vi "MP-285 Get Position.vi"(5 "error in (no error)":errorcluster, 6 "VISA resource name":refnum<visa-resource-name>) -> (0 "error out":errorcluster, 1 "Output: Z axis (microns)":dbl format="%.2f", 2 "Output: Y axis (microns)":dbl format="%.2f", 3 "Output: X axis (microns)":dbl format="%.2f", 4 "VISA resource name out":refnum<visa-resource-name>)   [LabVIEW 2010]
uses:
  StageMG100204SutterMP285/StageMG100204SutterMP285.lvclass
panel:
  out "last element CR?":bool
  out "return count":u32
  out "Serial Read":string
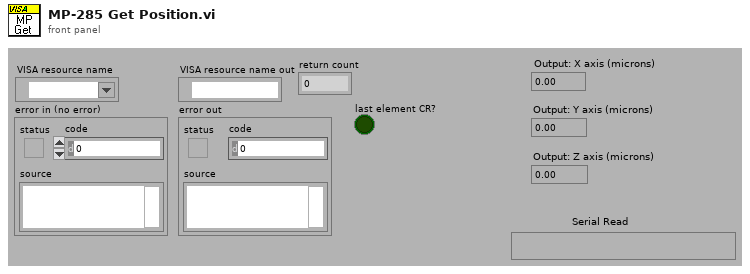
[diagram p1: front panel]
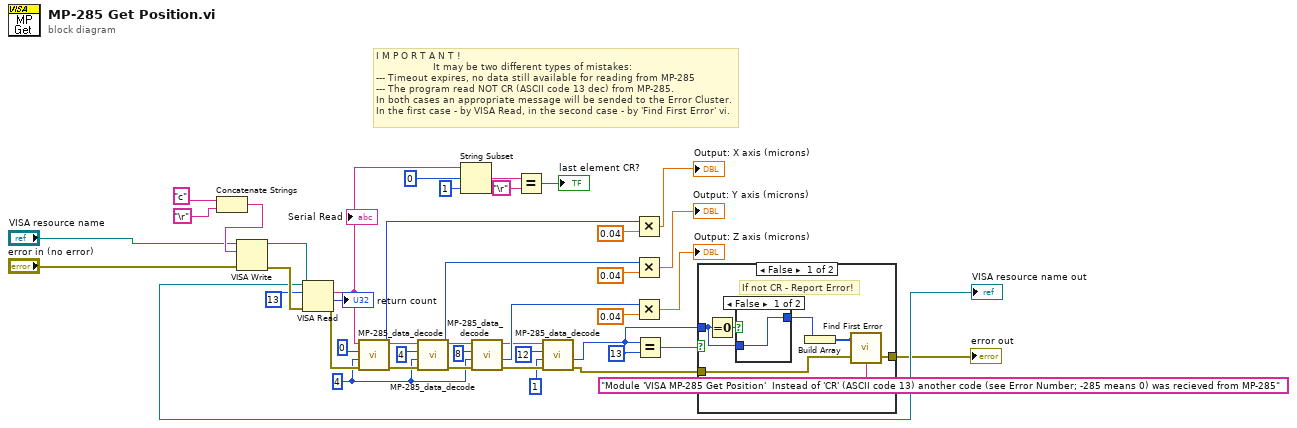
[diagram p0: block diagram]
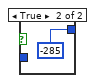
[diagram p2: hidden frame]
diagram:
  w9 = 4 ("length")
  # "I M P O R T A N T !\n                   It may be two different types of mistakes: \n--- Timeout expires, no data still available for reading from MP-285\n--- The program read NOT CR (ASCII code 13 dec) from MP-285.\nIn both cases an appropriate message will be sended to the Error Cluster.\nIn the first case - by VISA Read, in the second case - by 'Find First Error' vi."
  n1 = Concatenate Strings("c", "\r") -> (w32:string)
  n2 = VISA Write(VISA resource name="VISA resource name", write buffer=w32, error in (no error)="error in (no error)") -> (VISA resource name out=w31:refnum<visa-resource-name>, error out=w30:errorcluster)  [unwired: 1 out]
  n3 = VISA Read(VISA resource name=w31, byte count=u32 13, error in (no error)=w30) -> (VISA resource name out=→"VISA resource name out":refnum<visa-resource-name>, read buffer=w6:string, return count=→"return count":u32, error out=w15:errorcluster)
  "Serial Read" <- w6
  n4 = call "MP-285_data_decode.vi"("error in (no error)"=w15, "length"=w9, "offset"=0 ("offset (0)"), "encoded data string in"=w6) -> ("error out"=w14:errorcluster, "decoded data"=w40:i32)  [unwired: 5 in, 1 out]
  n5 = call "MP-285_data_decode.vi"("error in (no error)"=w14, "length"=w9, "offset"=4 ("length"), "encoded data string in"=w6) -> ("error out"=w13:errorcluster, "decoded data"=w36:i32)  [unwired: 5 in, 1 out]
  n6 = String Subset(string=w6, offset (0)=0, length (rest)=1 ("length (rest)")) -> (substring=w4:string)
  n7 = call "MP-285_data_decode.vi"("error in (no error)"=w13, "length"=w9, "offset"=8 ("offset (0)"), "encoded data string in"=w6) -> ("error out"=w12:errorcluster, "decoded data"=w37:i32)  [unwired: 5 in, 1 out]
  n8 = Equal?(x=w4, y="\r") -> (x = y?=→"last element CR?":bool)
  n9 = call "MP-285_data_decode.vi"("error in (no error)"=w12, "length"=1, "offset"=12, "encoded data string in"=w6) -> ("error out"=w17:errorcluster, "decoded data"=w23:i32)  [unwired: 5 in, 1 out]
  n10 = Multiply(x=w40, y=0.04) -> (x*y=→"Output: X axis (microns)":dbl)
  n11 = Multiply(x=w36, y=0.04) -> (x*y=→"Output: Y axis (microns)":dbl)
  n12 = Multiply(x=w37, y=0.04) -> (x*y=→"Output: Z axis (microns)":dbl)
  n13 = Equal?(x=w23, y=13) -> (x = y?=w24:bool)
  n14 = case shown="False" w24 {
    tunnel: [w47 w50] -> w18
    tunnel: w23 -> [w42 _]
    tunnel: w17 -> [w44 w50]
    frame False {
      # "If not CR - Report Error!"
      n15 = Equal To 0?(x=w42) -> (x = 0?=w43:bool)
      n16 = case shown="False" w43 {
        tunnel: w42 -> [w48 _]
        tunnel: [w48 -285] -> w41
        frame False {
        }
        frame True {
        }
      }
      n17 = Build Array(w41) -> (w45:i32[])
      n18 = call <vilib>:"Find First Error.vi"("error in (no error)"=w44, "source messages"="Module 'VISA MP-285 Get Position'  Instead of 'CR' (ASCII code 13) another code (see Error Number; -285 means 0) was recieved from MP-285", "error codes"=w45) -> ("error out"=w47:errorcluster)  [unwired: 2 out]
    }
    frame True {
      # "The CR was readed\n        NO Errors"
      # "TRUE CR was received - NO Errors"
    }
  }
  "error out" <- w18
